vi "Update Device Temperature(old).vi"(8 "error in (no error)":errorcluster, 10 "Data Cluster":T1, 11 "Message Queue in":refnum<class "Delacor_lib_QMH_Message Queue.lvclass">) -> (0 "error out":errorcluster, 2 "Data Cluster out":T1)   [LabVIEW 2015, in "Tool Module.lvlib"]
doc: "<b>Note:</b> This VI was modified by the <b>Validate DQMH Module</b> tool to turn off automatic error handling."
uses:
  Tool Module.lvlib
  _STATUS Typedef--cluster.ctl
  _Inspection Limits cluster--typedef.ctl
  QC-X App/Libraries/Event Logger Library/Event Log/EventLog.lvclass
  Module Data--cluster.ctl
  <vilib>/Delacor/Delacor QMH/Libraries/Message Queue_class/Delacor_lib_QMH_Message Queue.lvclass
  _Sample Data Rtn Cluster--typedef.ctl
  Tool Typedefs/_FPGA Timing Constraints Cluster--typedef.ctl
  Tool Typedefs/_FPGA Timing Ctrl Cluster--typedef.ctl
  Tool Typedefs/_FPGA Laser Config Cluster--typedef.ctl
  Tool Typedefs/_FPGA Peak Proc Cfg Cluster--typedef.ctl
  Tool Typedefs/_FPGA SPI Cfg Cluster--typedef.ctl
  Tool Typedefs/_FPGA Setup Params Cluster--typedef.ctl
  Return FPGA Setup Data (Reply Payload)--cluster.ctl
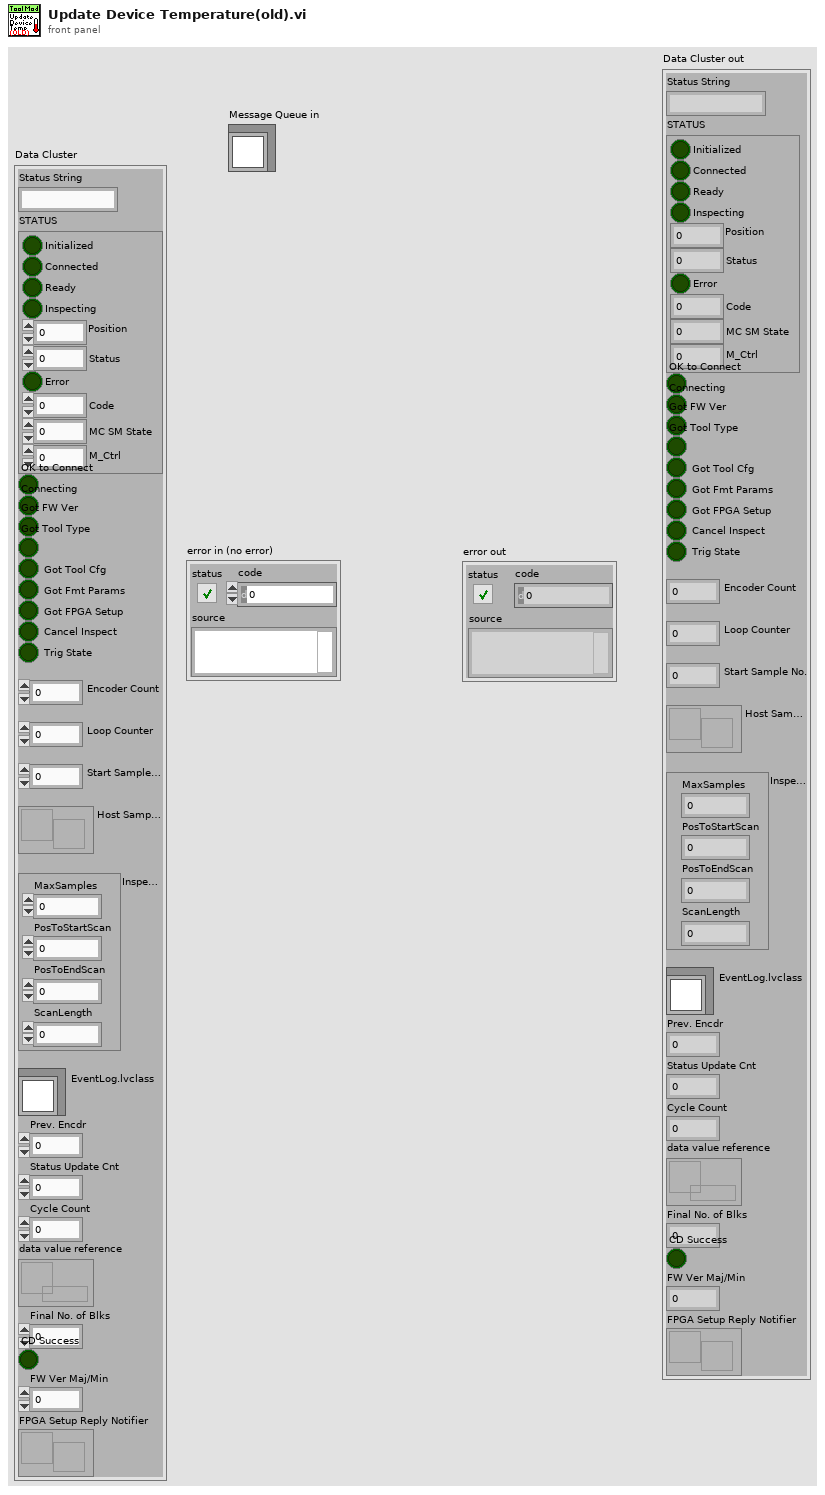
[diagram p1: front panel]
types:
  T1 = typedef "Tool Module.lvlib/Module Data--cluster.ctl" = cluster{"Status String":string, "STATUS":T2, "OK to Connect":bool, "Connecting":bool, "Got FW Ver":bool, "Got Tool Type":bool, "Got Tool Cfg":bool, "Got Fmt Params":bool, "Got FPGA Setup":bool, "Cancel Inspect":bool, "Trig State":bool, "Encoder Count":i32, "Loop Counter":i32, "Start Sample No.":u32, "Host SampleData":refnum<notifier>, "Inspection Limits":T3, "EventLog.lvclass":refnum<class "EventLog.lvclass">, "Prev. Encdr":i32, "Status Update Cnt":i32, "Cycle Count":i32, "data value reference":refnum<data-value>, "Final No. of Blks":i32, "CD Success":bool, "FW Ver Maj/Min":dbl, "FPGA Setup Reply Notifier":refnum<notifier>}
  T2 = typedef "Tool Module.lvlib/_STATUS Typedef--cluster.ctl" = cluster{"Initialized":bool, "Connected":bool, "Ready":bool, "Inspecting":bool, "Position":dbl, "Status":u16, "Error":bool, "Code":i32, "MC SM State":u16, "M_Ctrl":u16}
  T3 = typedef "Tool Module.lvlib/_Inspection Limits cluster--typedef.ctl" = cluster{"MaxSamples":i32, "PosToStartScan":i32, "PosToEndScan":i32, "ScanLength":i32}
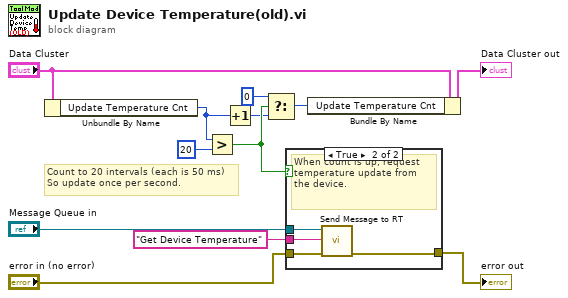
[diagram p0: block diagram]
diagram:
  # "Count to 20 intervals (each is 50 ms)\nSo update once per second."
  n1 = Unbundle By Name("Data Cluster") -> ("Update Temperature Cnt"=w5:i32)
  n2 = Greater?(x=w5, y=20) -> (0:w3:bool)
  n3 = Increment(x=w5) -> (x+1=w1:i32)
  n4 = Select(t=0, s=w3, f=w1) -> (s? t:f=w4:i32)
  n5 = case shown="True" w3 {
    tunnel: "Message Queue in" -> [_ w17]
    tunnel: "error in (no error)" -> [w13 w16]
    tunnel: "Get Device Temperature" ("Message") -> [_ w15]
    tunnel: [w13 w14] -> w2
    frame False {
    }
    frame True {
      # "When count is up, request temperature update from the device."
      n6 = call "Send Message to RT.vi"("error in (no error)"=w16, "Message"=w15, "Message Queue in"=w17) -> ("error out"=w14:errorcluster)  [unwired: 7 in, 1 out]
    }
  }
  "error out" <- w2
  n7 = Bundle By Name(cluster="Data Cluster", "Update Temperature Cnt"=w4) -> (→"Data Cluster out":T1)
